vi "pallet show.vi"(0 "Array":dbl[][](array[numeric]), 1 "palet num":i32, 2 "File Path":path, 3 "Image 2":T1, 5 "error in (no error)":errorcluster) -> (14 "This VI":refnum<vi>, 19 "error out":errorcluster)   [LabVIEW 2019]
uses:
  <vilib>/vision/Image Controls.llb/IMAQ Image.ctl
panel:
  out "GB sit":u32(colorbox)=16448250
  out "SYNC":bool
  out "Frm false":bool
  out "Pallet Analyzed":T1(plugin-control)
  out "SWL":bool
  out "SWR":bool
  out "PLT num":string="178"
  out "curv def":bool
  out "CURV":string
  out "GRBR":string="2"
  out "DEF type":string="1"
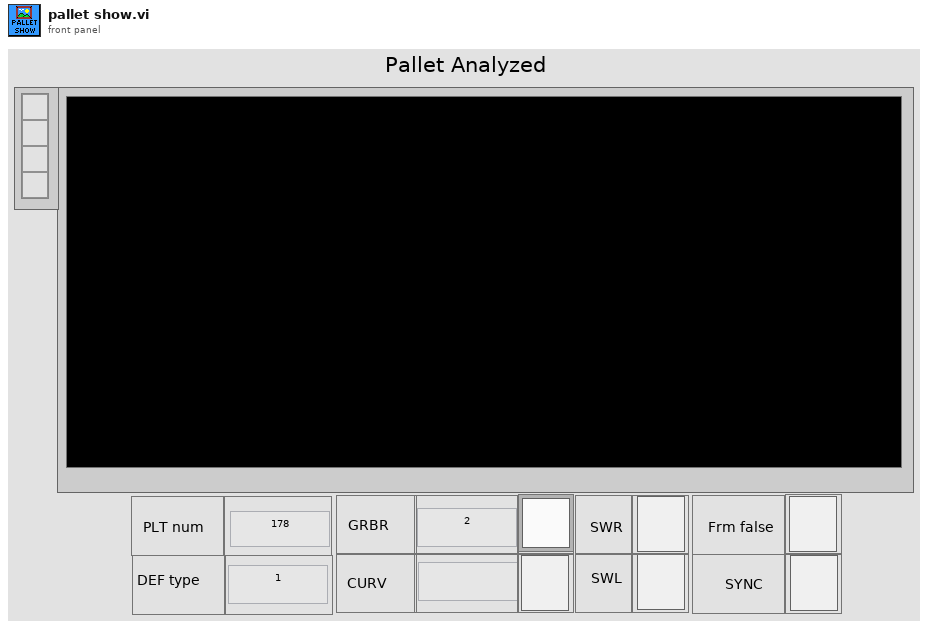
[diagram p1: front panel]
types:
  T1 = typedef "IMAQ Image.ctl" = refnum<image>
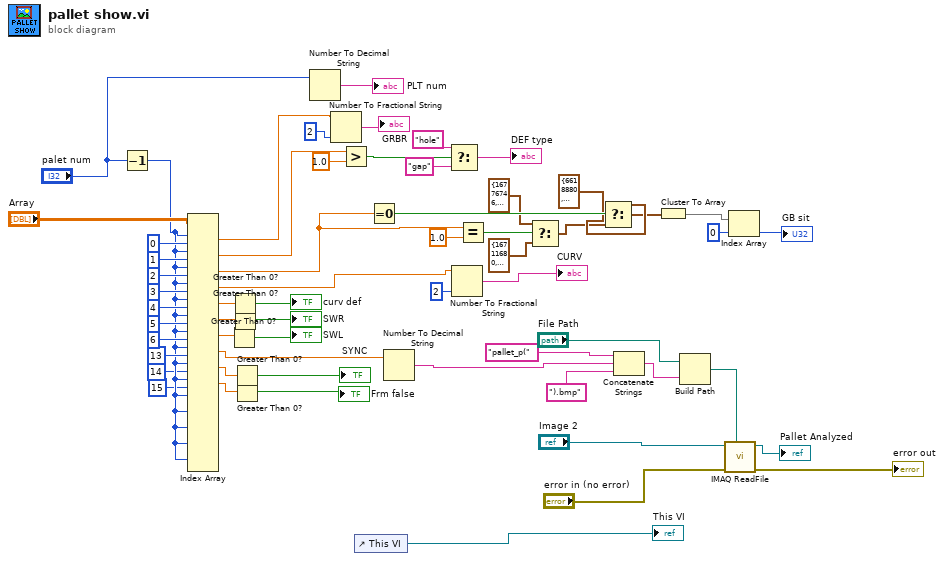
[diagram p0: block diagram]
diagram:
  n1 = Decrement(x="palet num") -> (x-1=w16:i32)
  n2 = Index Array(array="Array", index (row) #1=w16, index (col) #1=0 ("disabled index (col)"), index (row) #2=w16, index (col) #2=1 ("disabled index (col)"), index (row) #3=w16, index (col) #3=2 ("disabled index (col)"), index (row) #4=w16, index (col) #4=3 ("disabled index (col)"), index (row) #5=w16, index (col) #5=4 ("disabled index (col)"), index (row) #6=w16, index (col) #6=5 ("disabled index (col)"), index (row) #7=w16, index (col) #7=6 ("disabled index (col)"), index (row) #8=w16, index (col) #8=13 ("disabled index (col)"), index (row) #9=w16, index (col) #9=14 ("disabled index (col)"), index (row) #10=w16, index (col) #10=15 ("disabled index (col)"), index (row) #11=w16, index (row) #12=w16, index (row) #13=w16, index (row) #14=w16, index (row) #15=w16) -> (element #1=w7:dbl, element #2=w55:dbl, element #3=w47:dbl, element #4=w3:dbl, element #5=w32:dbl, element #6=w34:dbl, element #7=w33:dbl, element #8=w20:dbl, element #9=w11:dbl, element #10=w10:dbl)  [unwired: 5 in, 5 out]
  n3 = Greater Than 0?(x=w33) -> (x > 0?=→"SWL":bool)
  n4 = Greater Than 0?(x=w32) -> (x > 0?=→"curv def":bool)
  n5 = Greater Than 0?(x=w34) -> (x > 0?=→"SWR":bool)
  n6 = Greater Than 0?(x=w11) -> (x > 0?=→"SYNC":bool)
  n7 = Greater Than 0?(x=w10) -> (x > 0?=→"Frm false":bool)
  n8 = Number To Decimal String(number="palet num") -> (decimal integer string=→"PLT num":string)  [unwired: 1 in]
  n9 = Number To Fractional String(number=w7, precision (6)=i16 2 ("width (-)")) -> (F-format string=→"GRBR":string)  [unwired: 2 in]
  n10 = Greater?(x=w55, y=1.0) -> (0:w53:bool)
  n11 = control-ref of="This VI"() -> (→"This VI":refnum<vi>)
  n12 = Equal To 0?(x=w47) -> (x = 0?=w49:bool)
  n13 = Number To Decimal String(number=w20) -> (decimal integer string=w19:string)  [unwired: 1 in]
  n14 = Select(t="hole", s=w53, f="gap") -> (s? t:f=→"DEF type":string)
  n15 = Number To Fractional String(number=w3, precision (6)=i16 2) -> (F-format string=→"CURV":string)  [unwired: 2 in]
  n16 = Equal?(x=w47, y=1.0) -> (x = y?=w46:bool)
  n17 = Select(t=cluster{u32, u32} {16776746, 16776746} ("new element/subarray"), s=w46, f=cluster{u32, u32} {16711680, 16711680} ("new element/subarray")) -> (s? t:f=w43:cluster{u32, u32})
  n18 = Select(t=cluster{u32, u32} {6618880, 6618880} ("new element/subarray"), s=w49, f=w43) -> (s? t:f=w42:cluster{u32, u32})
  n19 = Concatenate Strings("pallet_p(" ("string"), w19, ").bmp" ("string")) -> (w21:string)
  n20 = Cluster To Array(cluster=w42) -> (array=w41:u32[])
  n21 = Build Path(base path="File Path", name or relative path=w21) -> (appended path=w24:path)
  n22 = call "IMAQ ReadFile"("File Path"=w24, "error in (no error)"="error in (no error)", "Image"="Image 2") -> ("error out"=→"error out":errorcluster, "Image Out"=→"Pallet Analyzed":T1)  [unwired: 4 in, 3 out]
  n23 = Index Array(array=w41, index=0) -> (element=→"GB sit":u32)
